vi "DrawImageWithAlphaChannel.vi"(7 "Alpha (255 opaque)":u8=255, 8 "Background Color":u32(colorbox)=16777215, 9 "Insertion Point (x,y)":cluster{"x":i16, "y":i16}, 10 "image data":T1, 11 "2D Picture in":picture) -> (3 "2D Picture out":picture)   [LabVIEW 2025, in "Picture2D.lvlib" / "Image.lvclass"]
uses:
  Image.lvclass
  <vilib>/picture/picture.llb/imagedata.ctl
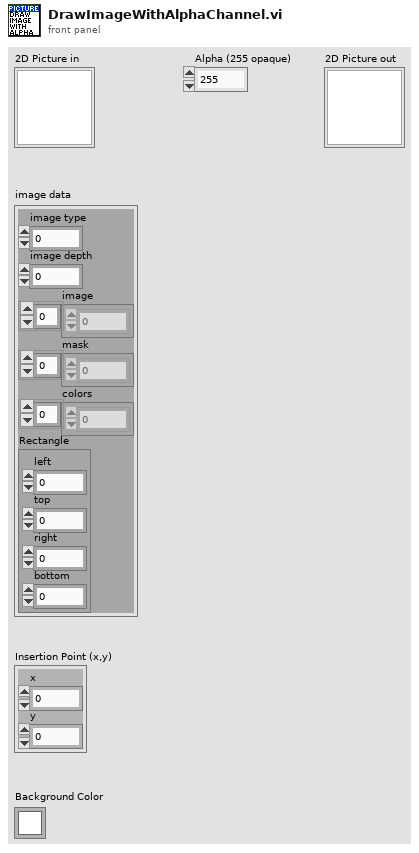
[diagram p1: front panel]
types:
  T1 = typedef "imagedata.ctl" = cluster{"image type":i32, "image depth":i32, "image":u8[], "mask":u8[], "colors":u32[], "Rectangle":cluster{"left":i16, "top":i16, "right":i16, "bottom":i16}}
  T2 = cluster{"left":i16, "top":i16, "right":i16, "bottom":i16}
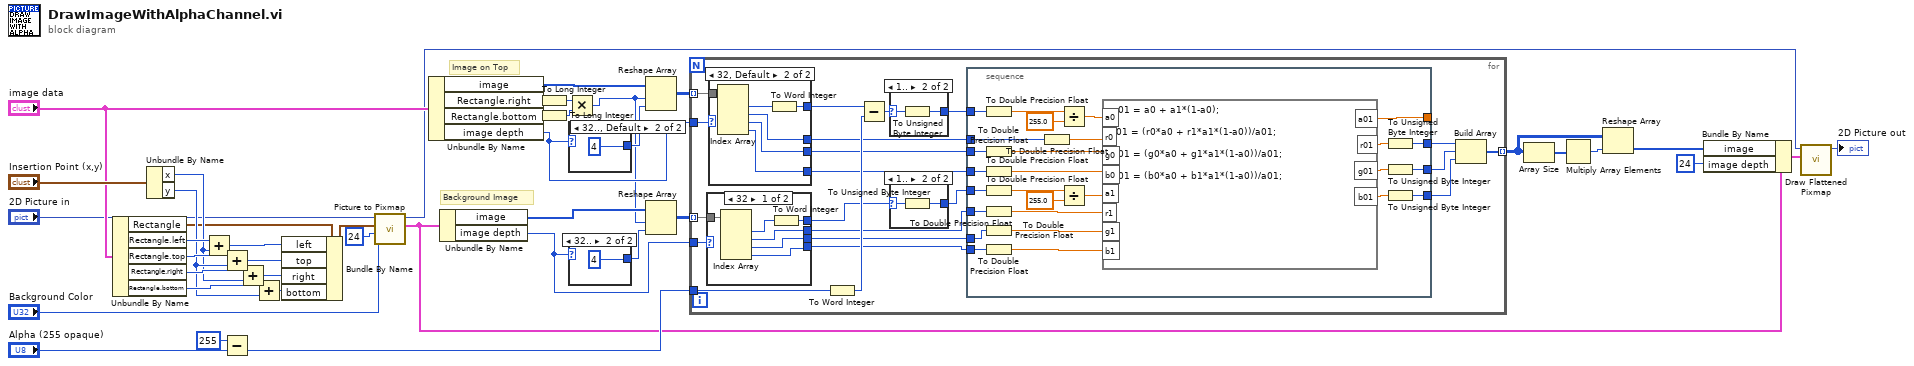
[diagram p0: block diagram]
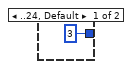
[diagram p2: hidden frame]
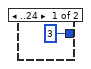
[diagram p3: hidden frame]
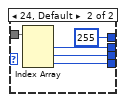
[diagram p4: hidden frame]
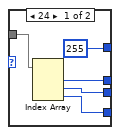
[diagram p5: hidden frame]
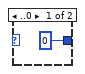
[diagram p6: hidden frame]
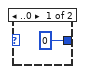
[diagram p7: hidden frame]
diagram:
  # "Image on Top"
  # "Background Image"
  n1 = Unbundle By Name("image data") -> ("Rectangle"=w8:T2, "Rectangle.left"=w32:i16, "Rectangle.top"=w34:i16, "Rectangle.right"=w35:i16, "Rectangle.bottom"=w36:i16)
  n2 = Unbundle By Name("Insertion Point (x,y)") -> ("x"=w30:i16, "y"=w31:i16)
  n3 = Add(x=w32, y=w30) -> (x+y=w33:i16)
  n4 = Add(x=w34, y=w31) -> (x+y=w39:i16)
  n5 = Subtract(x=u8 255, y="Alpha (255 opaque)") -> (x-y=w41:u8)
  n6 = Add(x=w35, y=w30) -> (x+y=w38:i16)
  n7 = Add(x=w36, y=w31) -> (x+y=w37:i16)
  n8 = Bundle By Name(cluster=w8, "left"=w33, "top"=w39, "right"=w38, "bottom"=w37) -> (w28:T2)
  n9 = call <vilib>:"Picture to Pixmap.vi"("Background Color"="Background Color", "depth"=24, "rect"=w28, "picture"="2D Picture in") -> ("image data"=w27:T1, "new picture"=w11:picture)  [unwired: 6 in]
  n10 = Unbundle By Name("image data") -> ("image"=w6:u8[], "Rectangle.right"=w4:i16, "Rectangle.bottom"=w5:i16, "image depth"=w24:i32)
  n11 = Unbundle By Name(w27) -> ("image"=w9:u8[], "image depth"=w25:i32)
  n12 = To Long Integer(number=w4) -> (32bit integer=w2:i32)
  n13 = To Long Integer(number=w5) -> (32bit integer=w1:i32)
  n14 = Multiply(x=w2, y=w1) -> (x*y=w3:i32)
  n15 = case shown="32.., Default" w24 {
    tunnel: [3 ("dimension size") 4 ("dimension size")] -> w21
    frame ..24 {
    }
    frame 32.., Default {
    }
  }
  n16 = case shown="32.." w25 {
    tunnel: [3 ("dimension size") 4 ("dimension size")] -> w22
    frame ..24, Default {
    }
    frame 32.. {
    }
  }
  n17 = Reshape Array(w6, w3, w21) -> (w7:u8[][])
  n18 = Reshape Array(w9, w3, w22) -> (w10:u8[][])
  n19 = for {
    tunnel: w7 -> [w67] mode=indexing
    tunnel: w10 -> [w66] mode=indexing
    tunnel: [w65] -> w17 mode=indexing
    tunnel: w41 -> [w64]
    tunnel: w24 -> [w50]
    tunnel: w25 -> [w49]
    n20 = case shown="32" w49 {
      tunnel: w66 -> [w73 w78]
      tunnel: [w72 w77] -> w56
      tunnel: [w71 w76] -> w55
      tunnel: [w70 w75] -> w54
      tunnel: [w68 i16 255] -> w48
      frame 32 {
        n21 = Index Array(array=w73) -> (element #1=w69:u8, element #2=w72:u8, element #3=w71:u8, element #4=w70:u8)  [unwired: 4 in]
        n22 = To Word Integer(number=w69) -> (16bit integer=w68:i16)
      }
      frame 24, Default {
        n23 = Index Array(array=w78) -> (element #1=w77:u8, element #2=w76:u8, element #3=w75:u8)  [unwired: 3 in]
      }
    }
    n24 = case shown="32, Default" w50 {
      tunnel: w67 -> [w80 w89]
      tunnel: [i16 255 w87] -> w60
      tunnel: [w83 w86] -> w59
      tunnel: [w82 w85] -> w58
      tunnel: [w81 w84] -> w57
      frame 24 {
        n25 = Index Array(array=w80) -> (element #1=w83:u8, element #2=w82:u8, element #3=w81:u8)  [unwired: 3 in]
      }
      frame 32, Default {
        n26 = Index Array(array=w89) -> (element #1=w88:u8, element #2=w86:u8, element #3=w85:u8, element #4=w84:u8)  [unwired: 4 in]
        n27 = To Word Integer(number=w88) -> (16bit integer=w87:i16)
      }
    }
    n28 = To Word Integer(number=w64) -> (16bit integer=w61:i16)
    n29 = Subtract(x=w60, y=w61) -> (x-y=w63:i16)
    n30 = case shown="1.." w63 {
      selector: w63 -> [_ w122]
      tunnel: [u8 0 w121] -> w62
      frame ..0 {
      }
      frame 1.. {
        n31 = To Unsigned Byte Integer(number=w122) -> (unsigned 8bit integer=w121:u8)
      }
    }
    n32 = case shown="1.." w48 {
      selector: w48 -> [_ w92]
      tunnel: [u8 0 w91] -> w47
      frame ..0 {
      }
      frame 1.. {
        n33 = To Unsigned Byte Integer(number=w92) -> (unsigned 8bit integer=w91:u8)
      }
    }
    n34 = stacked-sequence {
      tunnel: w47 -> [w119]
      tunnel: w62 -> [w118]
      tunnel: w59 -> [w117]
      tunnel: w58 -> [w116]
      tunnel: w57 -> [w115]
      tunnel: w56 -> [w114]
      tunnel: w55 -> [w113]
      tunnel: w54 -> [w112]
      tunnel: [w111] -> w53
      tunnel: [w110] -> w52
      tunnel: [w109] -> w51
      tunnel: [w93] -> _
      frame #0 {
        n35 = To Double Precision Float(number=w118) -> (double precision float=w99:dbl)
        n36 = To Double Precision Float(number=w116) -> (double precision float=w104:dbl)
        n37 = To Double Precision Float(number=w115) -> (double precision float=w103:dbl)
        n38 = To Double Precision Float(number=w119) -> (double precision float=w95:dbl)
        n39 = To Double Precision Float(number=w114) -> (double precision float=w102:dbl)
        n40 = To Double Precision Float(number=w113) -> (double precision float=w101:dbl)
        n41 = To Double Precision Float(number=w112) -> (double precision float=w100:dbl)
        n42 = To Double Precision Float(number=w117) -> (double precision float=w105:dbl)
        n43 = Divide(x=w99, y=255.0) -> (x/y=w98:dbl)
        n44 = Divide(x=w95, y=255.0) -> (x/y=w94:dbl)
        n45 = formula code="a01 = a0 + a1*(1-a0);\n\nr01 = (r0*a0 + r1*a1*(1-a0))/a01;\n\ng01 = (g0*a0 + g1*a1*(1-a0))/a01;\n\nb01 = (b0*a0 + b1*a1*(1-a0))/a01;"("a0"=w98, "r0"=w105, "r1"=w102, "g0"=w104, "g1"=w101, "b0"=w103, "b1"=w100, "a1"=w94) -> ("r01"=w108:dbl, "g01"=w107:dbl, "b01"=w106:dbl, "a01"=w93:dbl)
        n46 = To Unsigned Byte Integer(number=w108) -> (unsigned 8bit integer=w111:u8)
        n47 = To Unsigned Byte Integer(number=w107) -> (unsigned 8bit integer=w110:u8)
        n48 = To Unsigned Byte Integer(number=w106) -> (unsigned 8bit integer=w109:u8)
      }
    }
    n49 = Build Array(w53, w52, w51) -> (w65:u8[])
  }
  n50 = Array Size(array=w17) -> (size(s)=w18:i32[])
  n51 = Multiply Array Elements(1:w18) -> (0:w19:i32)
  n52 = Reshape Array(w17, w19) -> (w16:u8[])
  n53 = Bundle By Name(cluster=w27, "image"=w16, "image depth"=24) -> (w14:T1)
  n54 = call <vilib>:"Draw Flattened Pixmap.vi"("image data"=w14, "picture"=w11) -> ("new picture"=→"2D Picture out":picture)  [unwired: 7 in]
